vi "fault-reporting.vi"(0 "Path":path, 2 "Tower":bool, 3 "Condensor":bool, 4 "Cooler":bool, 5 "Air":bool, 6 "Converter":bool, 7 "Ammonia":bool) -> ()   [LabVIEW 2021]
uses:
  <vilib>/Utility/file.llb/Write Delimited Spreadsheet (string).vi
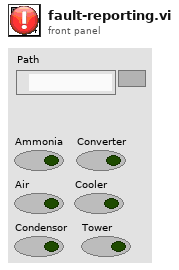
[diagram p1: front panel]
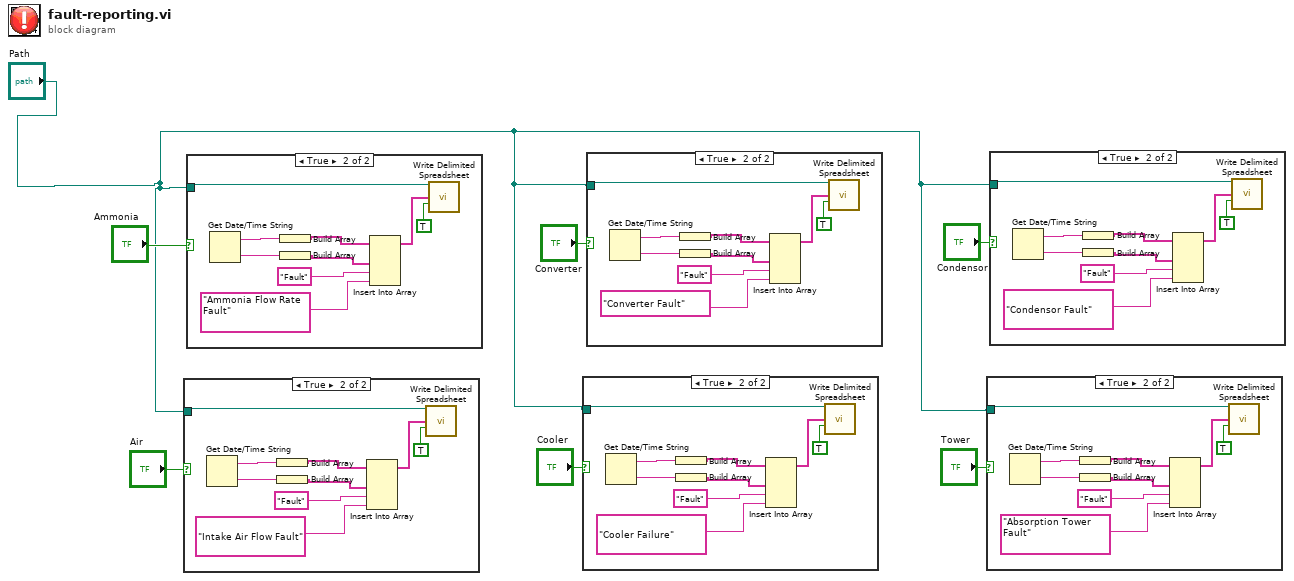
[diagram p0: block diagram]
diagram:
  n1 = case shown="True" "Air" {
    tunnel: "Path" -> [_ w8]
    frame False {
    }
    frame True {
      n2 = Get Date/Time String() -> (date string=w16:string, time string=w15:string)  [unwired: 3 in]
      n3 = Build Array(w16) -> (w14:string[])
      n4 = Build Array(w15) -> (w12:string[])
      n5 = Insert Into Array(array=w14, new element #1=w12, new element #2="Fault", new element #3="Intake Air Flow Fault") -> (w10:string[])  [unwired: 1 in]
      n6 = call-poly <vilib>:"Write Delimited Spreadsheet.vi"("file path (dialog if empty)"=w8, "1D data"=w10, "append to file? (new file:F)"=TRUE) -> ()  [unwired: 11 in, 2 out]
    }
  }
  n7 = case shown="True" "Ammonia" {
    tunnel: "Path" -> [_ w17]
    frame False {
    }
    frame True {
      n8 = Get Date/Time String() -> (date string=w25:string, time string=w24:string)  [unwired: 3 in]
      n9 = Build Array(w25) -> (w23:string[])
      n10 = Build Array(w24) -> (w21:string[])
      n11 = Insert Into Array(array=w23, new element #1=w21, new element #2="Fault", new element #3="Ammonia Flow Rate Fault") -> (w19:string[])  [unwired: 1 in]
      n12 = call-poly <vilib>:"Write Delimited Spreadsheet.vi"("file path (dialog if empty)"=w17, "1D data"=w19, "append to file? (new file:F)"=TRUE) -> ()  [unwired: 11 in, 2 out]
    }
  }
  n13 = case shown="True" "Cooler" {
    tunnel: "Path" -> [_ w26]
    frame False {
    }
    frame True {
      n14 = Get Date/Time String() -> (date string=w34:string, time string=w33:string)  [unwired: 3 in]
      n15 = Build Array(w34) -> (w32:string[])
      n16 = Build Array(w33) -> (w30:string[])
      n17 = Insert Into Array(array=w32, new element #1=w30, new element #2="Fault", new element #3="Cooler Failure") -> (w28:string[])  [unwired: 1 in]
      n18 = call-poly <vilib>:"Write Delimited Spreadsheet.vi"("file path (dialog if empty)"=w26, "1D data"=w28, "append to file? (new file:F)"=TRUE) -> ()  [unwired: 11 in, 2 out]
    }
  }
  n19 = case shown="True" "Converter" {
    tunnel: "Path" -> [_ w35]
    frame False {
    }
    frame True {
      n20 = Get Date/Time String() -> (date string=w43:string, time string=w42:string)  [unwired: 3 in]
      n21 = Build Array(w43) -> (w41:string[])
      n22 = Build Array(w42) -> (w39:string[])
      n23 = Insert Into Array(array=w41, new element #1=w39, new element #2="Fault", new element #3="Converter Fault") -> (w37:string[])  [unwired: 1 in]
      n24 = call-poly <vilib>:"Write Delimited Spreadsheet.vi"("file path (dialog if empty)"=w35, "1D data"=w37, "append to file? (new file:F)"=TRUE) -> ()  [unwired: 11 in, 2 out]
    }
  }
  n25 = case shown="True" "Tower" {
    tunnel: "Path" -> [_ w44]
    frame False {
    }
    frame True {
      n26 = Get Date/Time String() -> (date string=w52:string, time string=w51:string)  [unwired: 3 in]
      n27 = Build Array(w52) -> (w50:string[])
      n28 = Build Array(w51) -> (w48:string[])
      n29 = Insert Into Array(array=w50, new element #1=w48, new element #2="Fault", new element #3="Absorption Tower Fault") -> (w46:string[])  [unwired: 1 in]
      n30 = call-poly <vilib>:"Write Delimited Spreadsheet.vi"("file path (dialog if empty)"=w44, "1D data"=w46, "append to file? (new file:F)"=TRUE) -> ()  [unwired: 11 in, 2 out]
    }
  }
  n31 = case shown="True" "Condensor" {
    tunnel: "Path" -> [_ w53]
    frame False {
    }
    frame True {
      n32 = Get Date/Time String() -> (date string=w61:string, time string=w60:string)  [unwired: 3 in]
      n33 = Build Array(w61) -> (w59:string[])
      n34 = Build Array(w60) -> (w57:string[])
      n35 = Insert Into Array(array=w59, new element #1=w57, new element #2="Fault", new element #3="Condensor Fault") -> (w55:string[])  [unwired: 1 in]
      n36 = call-poly <vilib>:"Write Delimited Spreadsheet.vi"("file path (dialog if empty)"=w53, "1D data"=w55, "append to file? (new file:F)"=TRUE) -> ()  [unwired: 11 in, 2 out]
    }
  }
